vi "SendCmd_Tool.vi"(5 "path_bat":path=path "C:/Users/user/Desktop/tool/5.bat", 7 "error in (no error) 2":errorcluster) -> (2 "Accel_XYZ":string, 3 "HD Version":string, 4 "return code":i32, 6 "Other":string, 8 "release version:":string, 10 "Led Test":string, 13 "Gyro_XYZ":string, 14 "error out 3":errorcluster, 15 "version info":string)   [LabVIEW 2017]
panel:
  out "standard output":string
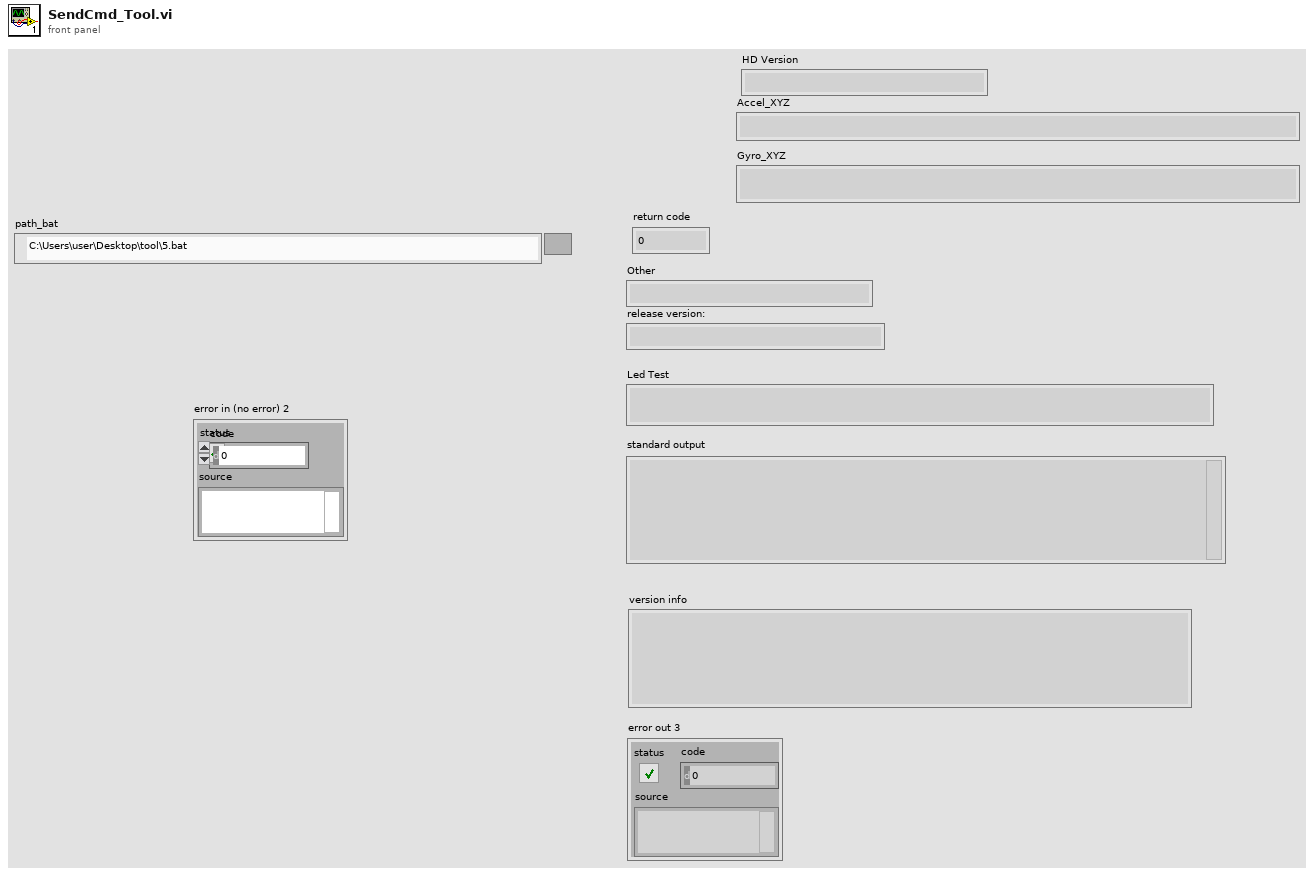
[diagram p1: front panel]
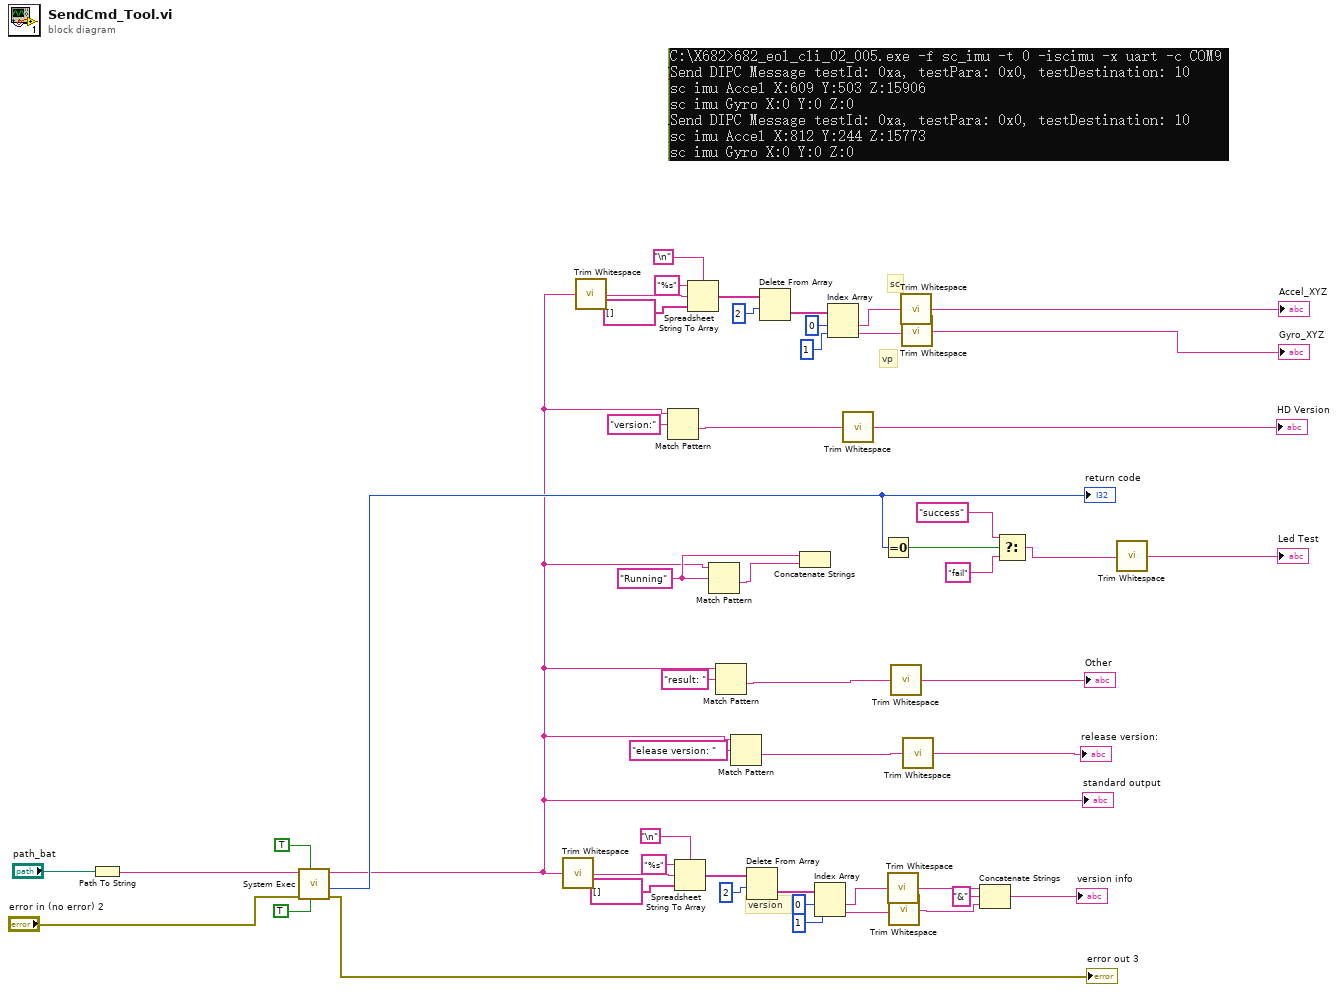
[diagram p0: block diagram]
diagram:
  w29 = "Running" ("regular expression")
  # "vp"
  # "sc"
  # "version"
  n1 = Path To String(path="path_bat") -> (string=w50:string)
  n2 = call <vilib>:"System Exec.vi"("run minimized? (F)"=TRUE, "wait until completion? (T)"=TRUE, "error in (no error)"="error in (no error) 2", "command line"=w50) -> ("error out"=→"error out 3":errorcluster, "return code"=w22:i32, "standard output"=w4:string)  [unwired: 2 in, 3 out]
  "return code" <- w22
  "standard output" <- w4
  n3 = call <vilib>:"Trim Whitespace.vi"("string"=w4) -> ("trimmed string"=w43:string)  [unwired: 1 in]
  n4 = call <vilib>:"Trim Whitespace.vi"("string"=w4) -> ("trimmed string"=w8:string)  [unwired: 1 in]
  n5 = Match Pattern(string=w4, regular expression="version:") -> (after substring=w16:string)  [unwired: 1 in, 3 out]
  n6 = Spreadsheet String To Array(delimiter (Tab)="\n", format string="%s", spreadsheet string=w43, array type (2D Dbl)=string[] []) -> (array=w42:string[])
  n7 = Spreadsheet String To Array(delimiter (Tab)="\n", format string="%s", spreadsheet string=w8, array type (2D Dbl)=string[] []) -> (array=w9:string[])
  n8 = Match Pattern(string=w4, regular expression=w29) -> (after substring=w28:string)  [unwired: 1 in, 3 out]
  n9 = Match Pattern(string=w4, regular expression="result: ") -> (after substring=w26:string)  [unwired: 1 in, 3 out]
  n10 = Match Pattern(string=w4, regular expression="elease version: ") -> (after substring=w24:string)  [unwired: 1 in, 3 out]
  n11 = Delete From Array(array=w42, length=2 ("index")) -> (deleted portion=w40:string[])  [unwired: 1 in, 1 out]
  n12 = Delete From Array(array=w9, length=2 ("index")) -> (deleted portion=w11:string[])  [unwired: 1 in, 1 out]
  n13 = Concatenate Strings(w29, w28) -> ()  [unwired: 1 out]
  n14 = Index Array(array=w40, index #1=0 ("index"), index #2=1 ("index")) -> (element #1=w35:string, element #2=w33:string)
  n15 = Index Array(array=w11, index #1=0 ("index"), index #2=1 ("index")) -> (element #1=w13:string, element #2=w14:string)
  n16 = call <vilib>:"Trim Whitespace.vi"("string"=w16) -> ("trimmed string"=→"HD Version":string)  [unwired: 1 in]
  n17 = Equal To 0?(x=w22) -> (x = 0?=w21:bool)
  n18 = call <vilib>:"Trim Whitespace.vi"("string"=w35) -> ("trimmed string"=w34:string)  [unwired: 1 in]
  n19 = call <vilib>:"Trim Whitespace.vi"("string"=w33) -> ("trimmed string"=w32:string)  [unwired: 1 in]
  n20 = call <vilib>:"Trim Whitespace.vi"("string"=w26) -> ("trimmed string"=→"Other":string)  [unwired: 1 in]
  n21 = call <vilib>:"Trim Whitespace.vi"("string"=w13) -> ("trimmed string"=→"Accel_XYZ":string)  [unwired: 1 in]
  n22 = call <vilib>:"Trim Whitespace.vi"("string"=w14) -> ("trimmed string"=→"Gyro_XYZ":string)  [unwired: 1 in]
  n23 = call <vilib>:"Trim Whitespace.vi"("string"=w24) -> ("trimmed string"=→"release version:":string)  [unwired: 1 in]
  n24 = Concatenate Strings(w34, "&" ("string"), w32) -> (→"version info":string)
  n25 = Select(t="success" ("string"), s=w21, f="fail" ("string")) -> (s? t:f=w18:string)
  n26 = call <vilib>:"Trim Whitespace.vi"("string"=w18) -> ("trimmed string"=→"Led Test":string)  [unwired: 1 in]
